vi "coag pump.vi"(11 "plant flow [L/s]":dbl) -> (0 "In Range?":bool, 1 "coag dose [mg/L]":dbl, 2 "pump [V]":dbl, 3 "coagulant flow [mL/s]":dbl, 5 "rpm":dbl)   [LabVIEW 2019]
uses:
  ini.ctl
  Sensor buffer command.ctl
panel:
  in  "coagulant stock [g/L]":dbl=72.0
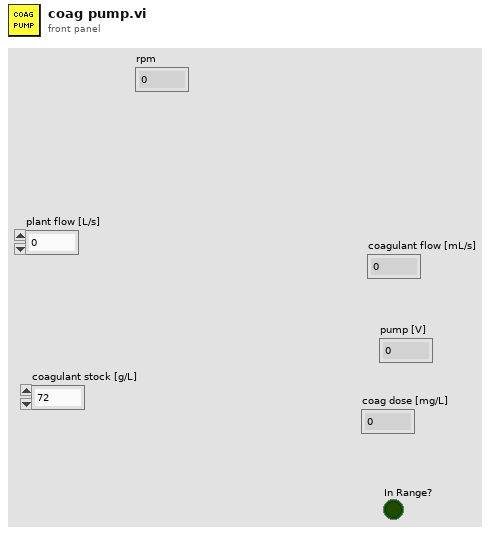
[diagram p1: front panel]
types:
  T1 = typedef "Sensor buffer command.ctl" = enum16{"set buffer size", "write", "refill buffer", "read recent", "read all", "read at delta HRT", "clear"}
  T2 = typedef "ini.ctl" = enum16{"write", "read"}
  T3 = typedef "data cluster.ctl" = cluster{"floc sed turbidity (NTU)":dbl, "Raw turbidity (NTU)":dbl, "flow rate (L/s)":dbl, "time":timestamp, "Cumulative HRT":dbl, "Coag dose (mg/L)":dbl, "DOM coag demand (mg/L)":dbl, "DOM in range":bool}
  T4 = typedef "setpoints.ctl" = cluster{"graph data interval (s)":sgl, "sludge flow [L/s]":dbl, "plant flow [L/s]":dbl, "Plant Flow PID ":cluster{"proportional gain (Kc)":dbl, "integral time (Ti, min)":dbl, "derivative time (Td, min)":dbl}, "Sludge PID ":cluster{"proportional gain (Kc)":dbl, "integral time (Ti, min)":dbl, "derivative time (Td, min)":dbl}, "backwash":T5, "Coagulant":T6}
  T5 = typedef "backwash.ctl" = cluster{"Filtered quality target [NTU]":dbl, "min filtration time [s]":dbl, "Ripen time [s]":dbl}
  T6 = typedef "coag.ctl" = cluster{"flocculator volume (L)":dbl, "clarifier volume (L)":dbl, "dose updates per response delay":u16, "target clarified turbidity (NTU)":dbl, "Coagulant mode":T7, "Coag dose [mg/L]":dbl, "pump mL/rev":dbl, "clarifier flow [L/s]":dbl, "min Coag dose [mg/L]":dbl, "max Coag dose [mg/L]":dbl, "Steps":u16, "HRT response delay":u32, "kpf":dbl, "DOM coag demand [mg/L]":dbl, "min DOM coag demand [mg/L]":dbl, "max DOM coag demand [mg/L]":dbl}
  T7 = typedef "model type.ctl" = enum16{"manual", "ramp", "simple corrector"}
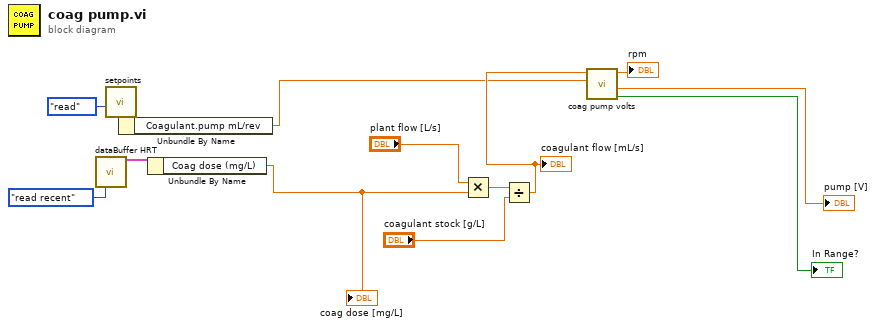
[diagram p0: block diagram]
diagram:
  n1 = call "dataBuffer HRT.vi"("command"=Sensor_buffer_command."read recent") -> ("recent data"=w2:T3)  [unwired: 9 in, 5 out]
  n2 = call "setpoints.vi"("ini"=ini."read") -> ("Setpoints out"=w9:T4)  [unwired: 9 in, 1 out]
  n3 = Unbundle By Name(w9) -> ("Coagulant.pump mL/rev"=w7:dbl)
  n4 = Unbundle By Name(w2) -> ("Coag dose (mg/L)"=w1:dbl)
  "coag dose [mg/L]" <- w1
  n5 = Multiply(x="plant flow [L/s]", y=w1) -> (x*y=w12:dbl)
  n6 = Divide(x=w12, y="coagulant stock [g/L]") -> (x/y=w8:dbl)
  "coagulant flow [mL/s]" <- w8
  n7 = call "coag pump volts.vi"("mL/rev"=w7, "coagulant flow [mL/s]"=w8) -> ("In Range?"=→"In Range?":bool, "V"=→"pump [V]":dbl, "rpm"=→"rpm":dbl)  [unwired: 7 in]
